vi "Destroy.vi"(8 "error in (no error)":errorcluster, 11 "reference in":refnum<class "Manipulator.lvclass">) -> (0 "error out":errorcluster, 3 "reference out":refnum<class "Manipulator.lvclass">)   [LabVIEW 2014, in "Manipulator.lvclass"]
uses:
  Manipulator.lvclass
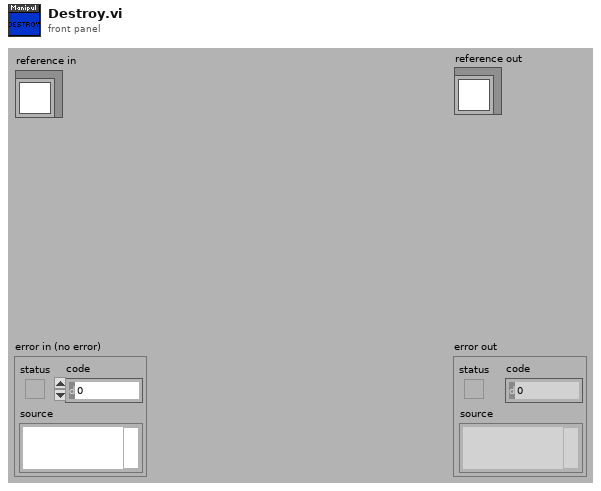
[diagram p1: front panel]
types:
  T1 = typedef "Manipulator.lvclass/ObjectAttributes.ctl" = cluster{"Coordinates":cluster{"X":dbl, "Y":dbl, "Z":dbl}, "Angles":cluster{"THETA_1":dbl, "THETA_2":dbl, "THETA_3":dbl, "THETA_4":dbl, "THETA_5":dbl, "THETA_6":dbl, "THETA_7":dbl, "THETA_8":dbl, "THETA_9":dbl, "THETA_10":dbl}, "Lengths":cluster{"a":dbl, "b":dbl, "c":dbl, "d":dbl, "e":dbl}, "Coordinates of joints":cluster{"A":cluster{"X":dbl, "Y":dbl, "Z":dbl}, "B":cluster{"X":dbl, "Y":dbl, "Z":dbl}, "C":cluster{"X":dbl, "Y":dbl, "Z":dbl}, "D":cluster{"X":dbl, "Y":dbl, "Z":dbl}}}
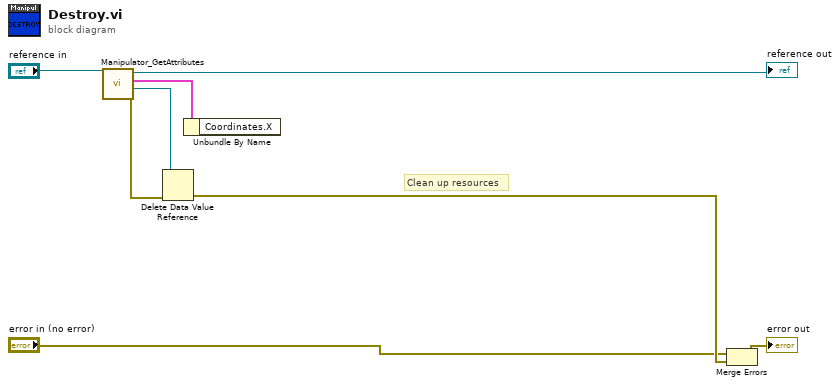
[diagram p0: block diagram]
diagram:
  # "Clean up resources"
  n1 = call "Manipulator_GetAttributes.vi"("reference in"="reference in") -> ("error out"=w5:errorcluster, "DataRef"=w4:refnum<data-value>, "Data"=w3:T1, "reference out"=→"reference out":refnum<class "Manipulator.lvclass">)  [unwired: 7 in]
  n2 = Delete Data Value Reference(data value reference=w4, error in=w5) -> (error out=w2:errorcluster)  [unwired: 1 out]
  n3 = Unbundle By Name(w3) -> ()  [unwired: 1 out]
  n4 = Merge Errors("error in (no error)", w2) -> (→"error out":errorcluster)
